vi "Main.vi"(7 "Panel":refnum<class "Panel.lvclass">, 11 "Module Admin":refnum<class "Delacor_lib_QMH_Module Admin.lvclass">) -> ()   [LabVIEW 2025, in "Chart.lvlib"]
doc: "This template is based from the Queued Message Handler design pattern and the Queued Message Handler Project Template that ships with LabVIEW 2014.\n\nThe main difference is that the Queue is private to this module and communication between modules is done via Broadcast and Request events.\n\nRequest events are wrapped via public API methods and are handled in the Event handler loop in this VI.\nAny module can register for Broadcast events sent by this module.\n\nThe Event Handling Loop generates messages based on user interface actions.\n\nThe Message Handling Loop processes messages generated by the Event Handling Loop, or by other messages. The messages are string values, so new messages can be added easily to the Message Cases case structure in the Message Handling Loop. Each message cluster can also provide an optional value for Message Data, which is a variant that can be converted to whatever message-specific data is required.\n_____\nBased on Delacor QMH Project Template 3.1.0.34.\n\n<b>Note:</b> This VI was modified by the <b>Validate DQMH Module</b> tool to call the Release Message Queue VI in the top-level Error case.\n\n<b>Note:</b> This VI was modified by the <b>Validate DQMH Module</b> tool to add a call to the Error Reported VI at the end of the 'Exit' MHL frame.\n\n<b>Note:</b> This VI was modified by the <b>Validate DQMH Module</b> tool to wrap the FP.Open method in the module close code with a Conditional Disable Structure so it does not execute when the Main VI is running as a built EXE."
uses:
  Chart.lvlib
  <vilib>/Delacor/Delacor QMH/Libraries/Module Admin_class/Delacor_lib_QMH_Module Admin.lvclass
  <vilib>/MGI/Panel Manager/Panel/Panel/Panel.lvclass
  <vilib>/Utility/miscctls.llb/LVPointTypeDef.ctl
  Module Data--cluster.ctl
  Initialise Chart Buffer Argument--cluster.ctl
  Update Chart Buffer Data Argument--cluster.ctl
  Update Chart Display Argument--cluster.ctl
  Set Chart Plot Labels Argument--cluster.ctl
  <vilib>/Delacor/Delacor QMH/Libraries/Module Admin_class/Delacor_lib_QMH_Module Admin.lvclass/Delacor_lib_QMH_Module Admin.ctl
  <vilib>/Delacor/Delacor QMH/Libraries/Message Queue_class/Delacor_lib_QMH_Message Queue.lvclass/Delacor_lib_QMH_Message Queue.ctl
  Stop Argument--cluster.ctl
  <vilib>/Delacor/Delacor QMH/Libraries/Message Queue_class/Delacor_lib_QMH_Enqueue Message (Single).vi
  <vilib>/Delacor/Delacor QMH/Libraries/Module Admin_class/Delacor_lib_QMH_Get External Launch.vi
  <vilib>/Utility/error.llb/Error Cluster From Error Code.vi
  <vilib>/ErrorRing/Error Ring.xnode
  <vilib>/Delacor/Delacor QMH/Libraries/Message Queue_class/Delacor_lib_QMH_Message Queue.lvclass
  <vilib>/MGI/Panel Manager/Panel/Panel Helper/Panel Helper.lvclass
panel:
  out "Waveform Graph":cluster{dbl, dbl, "Chart Data":dbl[][]}(graph)
  in  "Radio Buttons":enum32{"1 min", "10 min", "1 hr", "10 hr"}(radio)
  in  "Simulate MHL Error":bool
  in  "Simulate EHL Error":bool
  out "error out":errorcluster
  out "Status":string
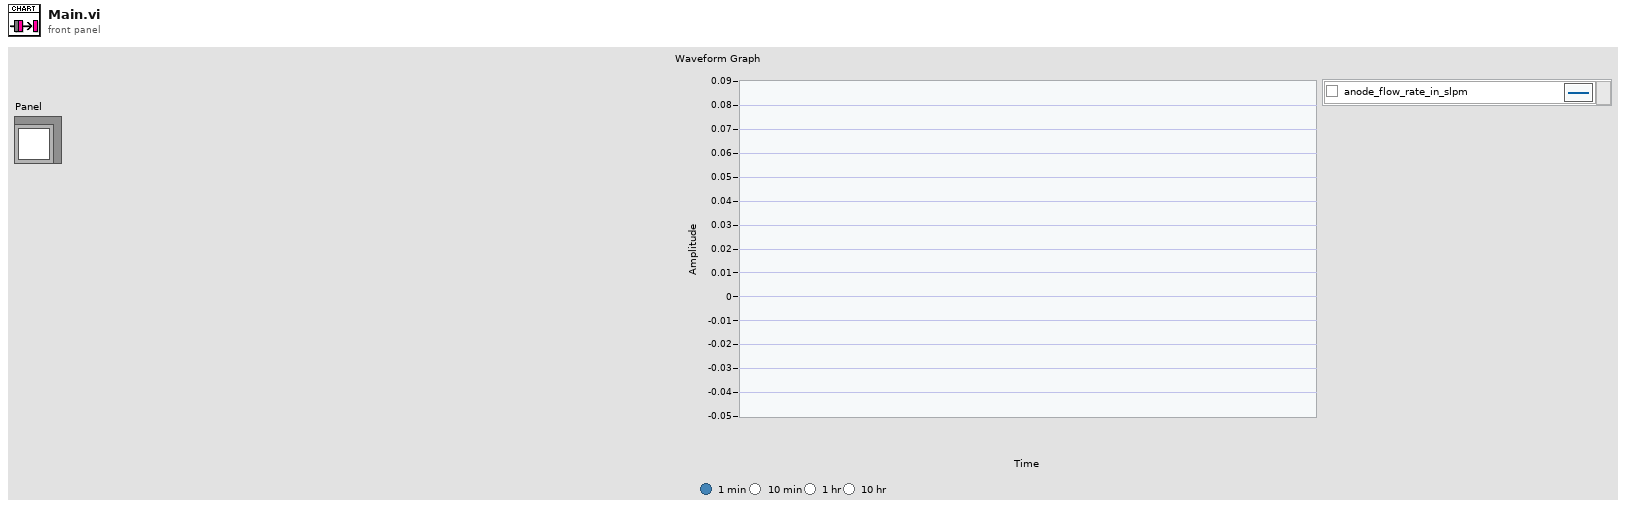
[diagram p1: front panel]
types:
  T1 = typedef "LVPointTypeDef.ctl" = cluster{"Horizontal":i16, "Vertical":i16}
  T2 = typedef "Chart.lvlib/Request Events--cluster.ctl" = cluster{"Stop Module":refnum<user-event>, "Show Panel":refnum<user-event>, "Hide Panel":refnum<user-event>, "Get Module Execution Status":refnum<user-event>, "Show Diagram":refnum<user-event>, "Change Panel":refnum<user-event>, "Initialise Chart Buffer":refnum<user-event>, "Update Chart Buffer Data":refnum<user-event>, "Update Chart Display":refnum<user-event>, "Set Chart Plot Labels":refnum<user-event>}
  T3 = typedef "Panel.lvlib/Panel Helper.lvclass/Panel Events.ctl" = cluster{"My Panel":refnum<user-event>, "Top Level Initialized":refnum<user-event>}
  T4 = typedef "Chart.lvlib/Module Data--cluster.ctl" = cluster{"Status":string, "Chart Index":i32, "Chart Data Array":dbl[][], "Frequency":dbl}
  T5 = typedef "Chart.lvlib/Stop Argument--cluster.ctl" = cluster{"Origin":string, "Exit via Stop Module Req?":bool, "Wait for Module to stop?":bool}
  T6 = typedef "Chart.lvlib/Initialise Chart Buffer Argument--cluster.ctl" = cluster{"No. of Channels":u32, "Frequency":dbl}
  T7 = typedef "Chart.lvlib/Update Chart Buffer Data Argument--cluster.ctl" = cluster{"Chart Data":dbl[]}
  T8 = typedef "Chart.lvlib/Update Chart Display Argument--cluster.ctl" = cluster{"Boolean":bool}
  T9 = typedef "Chart.lvlib/Set Chart Plot Labels Argument--cluster.ctl" = cluster{"Labels":string[]}
  T10 = enum32{"invalid lock state", "Not Locked", "Locked (No Password)", "Password-protected"}
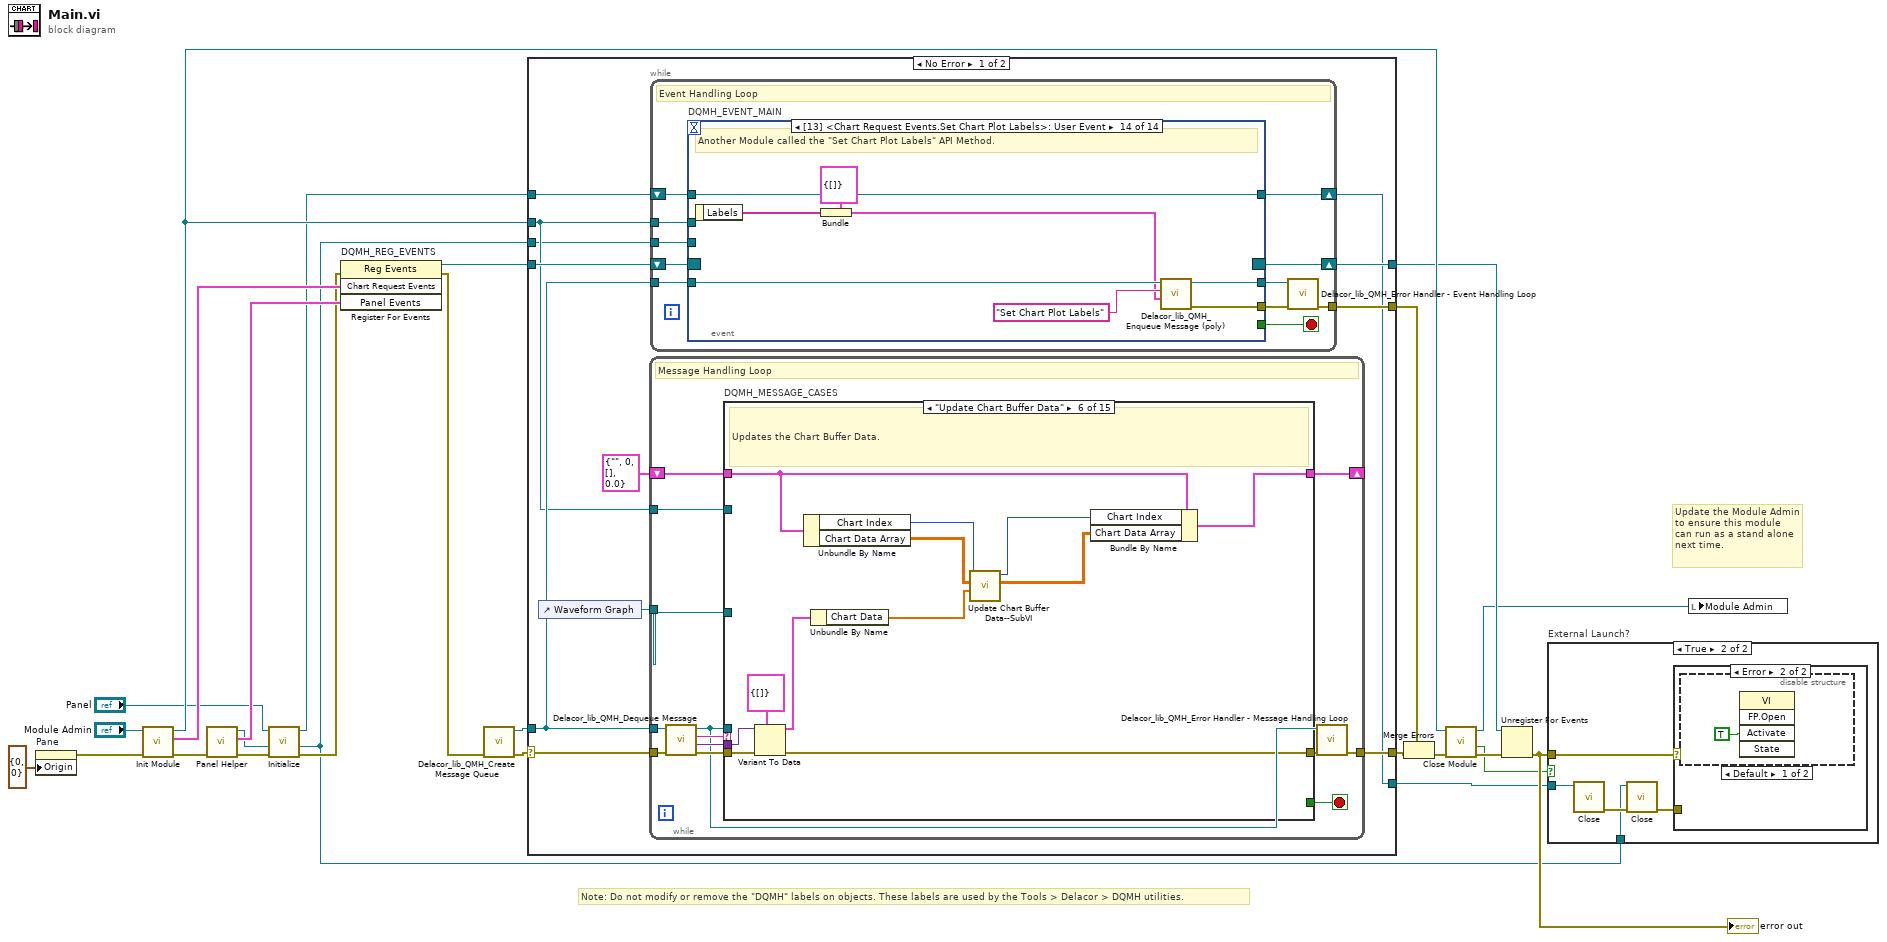
[diagram p0: block diagram]
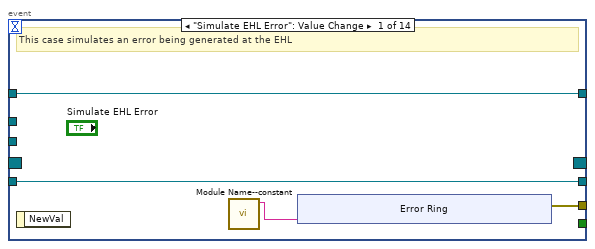
[diagram p5: hidden frame]
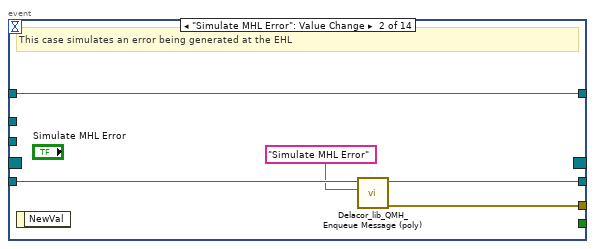
[diagram p6: hidden frame]
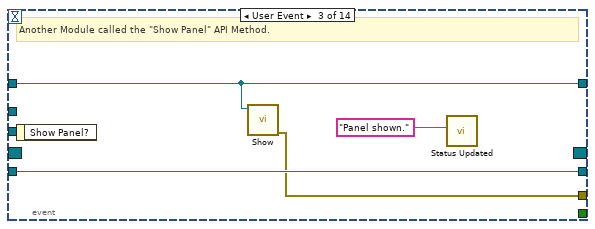
[diagram p7: hidden frame]
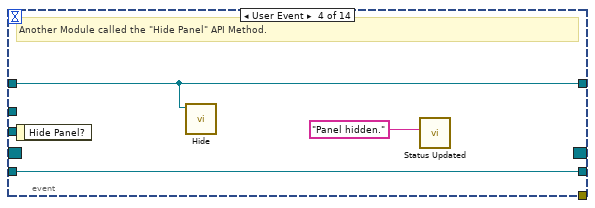
[diagram p8: hidden frame]
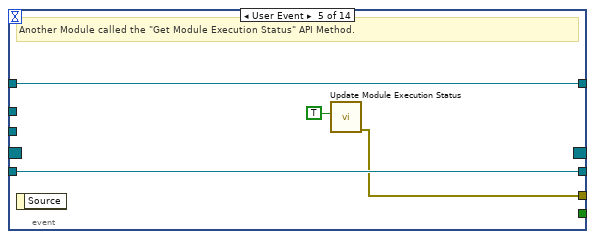
[diagram p9: hidden frame]
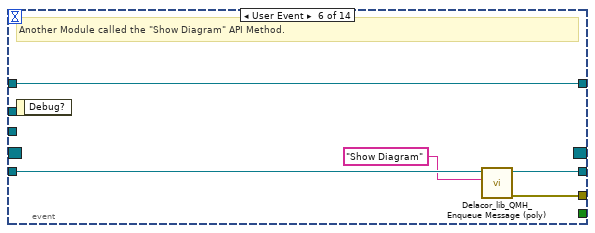
[diagram p10: hidden frame]
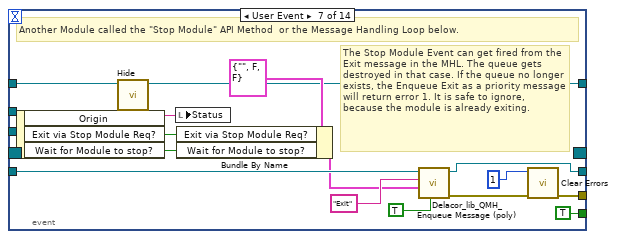
[diagram p11: hidden frame]
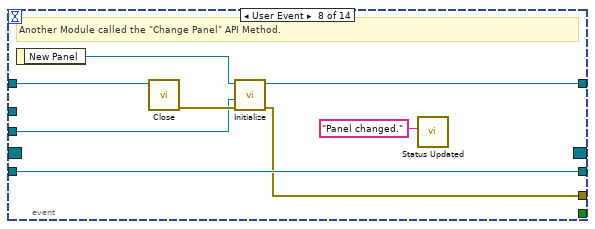
[diagram p12: hidden frame]
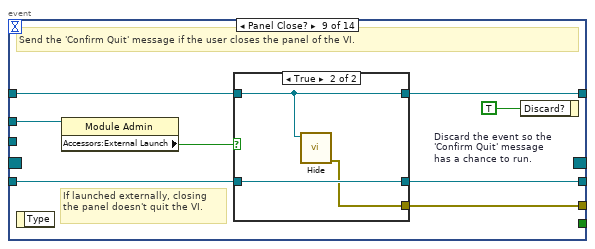
[diagram p13: hidden frame]
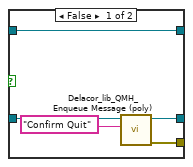
[diagram p14: hidden frame]
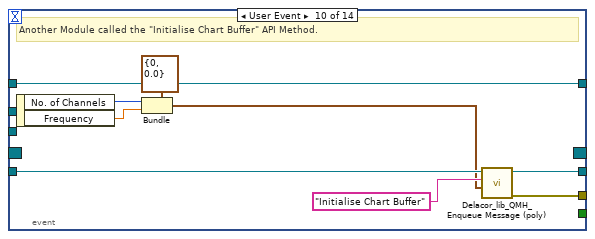
[diagram p15: hidden frame]
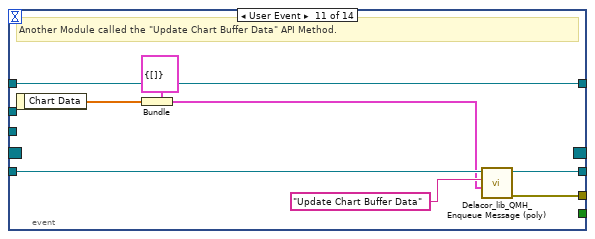
[diagram p16: hidden frame]
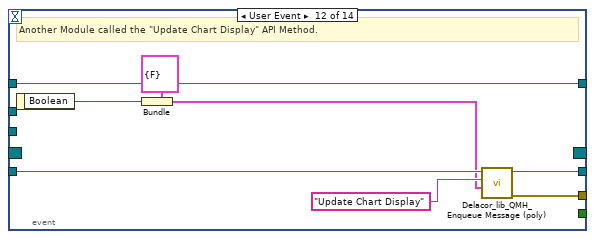
[diagram p17: hidden frame]
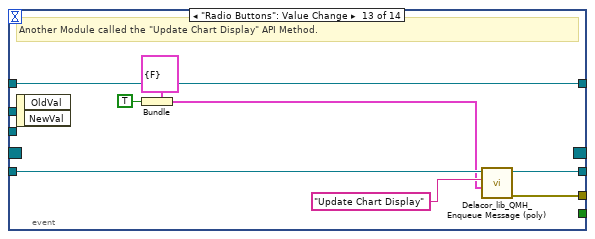
[diagram p18: hidden frame]
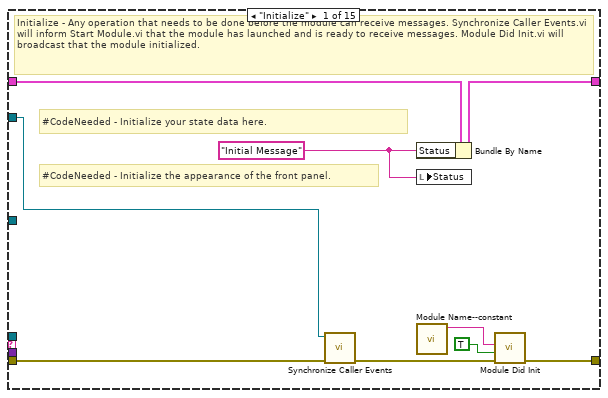
[diagram p19: hidden frame]
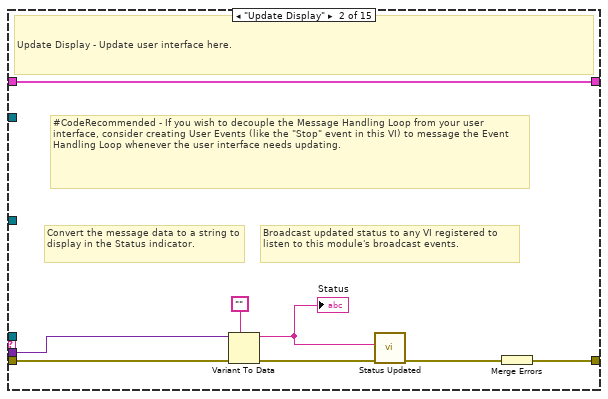
[diagram p20: hidden frame]
diagram:
  # "Note: Do not modify or remove the \"DQMH\" labels on objects. These labels are used by the Tools > Delacor > DQMH utilities."
  # "Update the Module Admin to ensure this module can run as a stand alone next time."
  n1 = property on="Pane" class="Pane"("Origin"=T1 {"Horizontal"=0, "Vertical"=0}) -> (error out=w1:errorcluster)  [unwired: 2 in, 1 out]
  n2 = call "Init Module.vi"("error in (no error)"=w1, "Singleton Module Admin in"="Module Admin") -> ("error out"=w11:errorcluster, "Chart Request Events"=w22:T2, "Singleton Module Admin out"=w26:refnum<class "Delacor_lib_QMH_Module Admin.lvclass">)  [unwired: 7 in]
  n3 = call <vilib>:"Panel Helper.vi"("Error In"=w11) -> ("Error Out"=w8:errorcluster, "Panel Events"=w10:T3, "Panel Helper out"=w7:refnum<class "Panel Helper.lvclass">)  [unwired: 8 in]
  n4 = call <vilib>:"Initialize.vi"("error in (no error)"=w8, "My Helper in"=w7, "Panel In"="Panel") -> ("error out"=w5:errorcluster, "My Helper out"=w4:refnum<class "Panel Helper.lvclass">, "Panel Out"=w3:refnum<class "Panel.lvclass">)  [unwired: 6 in]
  n5 = register-events "DQMH_REG_EVENTS"(error in=w5, w22, w10) -> (reference out=w23:refnum<event-registration>, error out=w9:errorcluster)  [unwired: 1 in]
  n6 = call <vilib>:"Delacor_lib_QMH_Create Message Queue.vi"("error in"=w9) -> ("error out"=w13:errorcluster, "Message Queue"=w21:refnum<class "Delacor_lib_QMH_Message Queue.lvclass">)  [unwired: 9 in]
  n7 = case shown="No Error" w13 {
    selector: w13 -> [w32 w363]
    tunnel: [w38 w363] -> w25
    tunnel: [w37 w368] -> w24
    tunnel: w23 -> [w35 w368]
    tunnel: w21 -> [w34 w359]
    tunnel: [w33 _] -> w17
    tunnel: w26 -> [w31 w364]
    tunnel: w3 -> [w29 w360]
    tunnel: w4 -> [w30 _]
    tunnel: [w28 w360] -> w12
    frame No Error {
      n8 = control-ref of="Waveform Graph"() -> (w27:refnum<vi>)
      n9 = while {
        tunnel: w34 -> [w165]
        shift-right: [w171] -> _
        shift-left: T4 {"Status"="", "Chart Index"=0, "Chart Data Array"=[], "Frequency"=0.0} ("Data Cluster") -> [w172]
        tunnel: w32 -> [w169]
        tunnel: [w163] -> w38
        tunnel: w31 -> [w162]
        tunnel: w27 -> [w161]
        stop <- w170 stop-if-true
        # "Message Handling Loop"
        n10 = call-dynamic "Delacor_lib_QMH_Dequeue Message.vi"("error in"=w169, "Message Queue in"=w165) -> ("error out"=w168:errorcluster, "Message Data"=w166:variant, "Message"=w167:string, "Message Queue out"=w164:refnum<class "Delacor_lib_QMH_Message Queue.lvclass">)  [unwired: 6 in]
        n11 = case "DQMH_MESSAGE_CASES" shown="\"Update Chart Buffer Data\"" w167 {
          selector: w167 -> [_ _ _ _ _ _ _ _ _ _ _ _ _ _ w348]
          tunnel: w164 -> [_ _ _ _ _ _ _ _ _ _ _ w313 w328 w344 _]
          tunnel: w168 -> [w174 w188 w192 w210 w224 w236 w256 w283 w294 w297 w302 w319 w332 w346 _]
          tunnel: [w177 w189 w191 w208 w223 w235 w255 w272 w292 w295 w300 w310 w330 w340 w349] -> w173
          tunnel: w172 -> [w182 w190 w193 w209 w212 w229 w242 w282 w293 w296 w301 w318 w331 w343 w350]
          tunnel: [w181 w190 w193 w209 w211 w228 w242 w282 w293 w296 w301 w318 w331 w343 w350] -> w171
          tunnel: [_ _ _ _ _ _ _ _ _ _ _ _ _ w342 _] -> w170
          tunnel: w166 -> [_ w187 _ _ w222 w234 w254 w281 _ _ _ w317 _ w339 _]
          tunnel: w162 -> [w175 _ _ _ _ _ _ _ _ _ _ w312 _ w333 _]
          tunnel: w161 -> [_ _ _ _ _ _ w237 w269 _ _ _ _ _ _ _]
          frame "Initialize" {
            w180 = "Initial Message" ("Initial Message")
            # "#CodeNeeded - Initialize the appearance of the front panel."
            # "#CodeNeeded - Initialize your state data here."
            # "Initialize - Any operation that needs to be done before the module can receive messages. Synchronize Caller Events.vi will inform Start Module.vi that the module has launched and is ready to receive messages. Module Did Init.vi will broadcast that the module initialized."
            n12 = call "Synchronize Caller Events.vi"("error in (no error)"=w174, "Singleton Module Admin in"=w175) -> ("error out"=w176:errorcluster)  [unwired: 8 in, 1 out]
            n13 = Bundle By Name(cluster=w182, "Status"=w180) -> (w181:T4)
            n14 = local write "Status"(w180) -> ()
            n15 = call "Module Name--constant.vi"() -> ("Module Name"=w178:string)  [unwired: 11 in]
            n16 = call "Module Did Init.vi"("error in (no error)"=w176, "Initialized?"=TRUE, "Origin"=w178) -> ("error out"=w177:errorcluster)  [unwired: 8 in]
          }
          frame "Update Display" {
            # "Broadcast updated status to any VI registered to listen to this module's broadcast events."
            # "Convert the message data to a string to display in the Status indicator."
            # "#CodeRecommended - If you wish to decouple the Message Handling Loop from your user interface, consider creating User Events (like the \"Stop\" event in this VI) to message the Event Handling Loop whenever the user interface needs updating."
            # "Update Display - Update user interface here."
            n17 = Variant To Data(error in=w188, type="" ("Empty String Constant"), Variant=w187) -> (data=w185:string, error out=w184:errorcluster)
            "Status" <- w185
            n18 = call "Status Updated.vi"("error in (no error)"=w184, "Status"=w185) -> ("error out"=w183:errorcluster)  [unwired: 9 in]
            n19 = Merge Errors(w183) -> (w189:errorcluster)
          }
          frame "Show Diagram" {
            # "Show Diagram - Show the block diagram of this VI. Used as a debugging tool. There is a button in the module tester that fires the Show Diagram request, which runs this message. Note that the diagram will not be displayed if it is password-protected and the password is not in the cache."
            n20 = disable-structure shown="RUN_TIME_ENGINE==False" {
              disable-tunnel: [w201 w207] -> w191
              disable-tunnel: w192 -> [w200 w207]
              frame condition #0 (active) {
                # "functionality not available in exe"
                n21 = invoke on="Invoke Node" class="VI" method="Lock State.Get"(error in=w200) -> (error out=w199:errorcluster, "Get Lock State"=w198:T10, "pwd in cache"=w195:bool)  [unwired: 3 in, 1 out]
                n22 = Equal?(x=T10."Password-protected", y=w198) -> (x = y?=w196:bool)
                n23 = Compound Arithmetic op=AND(w196, invert w195) -> (w194:bool)
                n24 = case shown="False" w194 {
                  tunnel: [w204 w206] -> w201
                  tunnel: w199 -> [w202 w206]
                  frame False {
                    n25 = property on="Property Node" class="VI"(error in=w202, "BDWin.Open"=TRUE ("Block Diagram Window:Open")) -> (error out=w204:errorcluster)  [unwired: 1 in, 1 out]
                    n26 = call "Status Updated.vi"("Status"="Block Diagram shown." ("format string")) -> ()  [unwired: 10 in, 1 out]
                  }
                  frame True {
                    # "Password-protected VI, and the password is not in the cache. Do not show the diagram."
                  }
                }
              }
              frame condition #1 {
              }
            }
          }
          frame "--- Module Specific ---" {
            # "Separator -- The following cases handle messages specific to this Module."
            n27 = Merge Errors(w210) -> (w208:errorcluster)
          }
          frame "Initialise Chart Buffer" {
            # "Initialises the chart buffer."
            n28 = Variant To Data(error in=w224, type=T6 {"No. of Channels"=0, "Frequency"=0.0} ("Initialise Chart Buffer Argument"), Variant=w222) -> (data=w213:T6, error out=w223:errorcluster)
            n29 = Unbundle By Name(w213) -> ("No. of Channels"=w215:u32, "Frequency"=w216:dbl)
            n30 = Multiply(x=w216, y=36000.0) -> (x*y=w214:dbl)
            n31 = Initialize Array(nan ("element"), w215, w214) -> (w217:dbl[][])
            n32 = Bundle By Name(cluster=w212, "Chart Index"=0, "Chart Data Array"=w217, "Frequency"=w216) -> (w211:T4)
          }
          frame "Update Chart Buffer Data" {
            # "Updates the Chart Buffer Data."
            n33 = Variant To Data(error in=w236, type=T7 {"Chart Data"=[]} ("Update Chart Buffer Data Argument"), Variant=w234) -> (data=w232:T7, error out=w235:errorcluster)
            n34 = Unbundle By Name(w229) -> ("Chart Index"=w226:i32, "Chart Data Array"=w231:dbl[][])
            n35 = Unbundle By Name(w232) -> ("Chart Data"=w230:dbl[])
            n36 = call "Update Chart Buffer Data--SubVI.vi"("Chart Data"=w230, "Chart Buffer In"=w231, "Chart Index In"=w226) -> ("Chart Buffer Out"=w227:dbl[][], "Chart Index Out"=w225:i32)  [unwired: 7 in]
            n37 = Bundle By Name(cluster=w229, "Chart Index"=w225, "Chart Data Array"=w227) -> (w228:T4)
          }
          frame "Update Chart Display" {
            # "Updates the Chart Display."
            n38 = Unbundle By Name(w242) -> ("Chart Data Array"=w246:dbl[][], "Chart Index"=w252:i32, "Frequency"=w250:dbl)
            n39 = Variant To Data(error in=w256, type=T8 {"Boolean"=FALSE} ("Update Chart Display Argument"), Variant=w254) -> (error out=w255:errorcluster)  [unwired: 1 out]
            n40 = Get Date/Time In Seconds() -> (seconds since 1Jan1904=w251:timestamp)
            n41 = case shown="\"10 hr\"" "Radio Buttons" {
              tunnel: w250 -> [w259 w262 w265 w268]
              tunnel: [w258 w261 w264 w267] -> w245
              tunnel: [w257 w260 w263 w266] -> w247
              frame "1 min", Default {
                w257 = 60.0 ("y")
                n42 = Multiply(x=w259, y=w257) -> (x*y=w258:dbl)
              }
              frame "10 min" {
                w260 = 600.0 ("y")
                n43 = Multiply(x=w262, y=w260) -> (x*y=w261:dbl)
              }
              frame "1 hr" {
                w263 = 3600.0 ("y")
                n44 = Multiply(x=w265, y=w263) -> (x*y=w264:dbl)
              }
              frame "10 hr" {
                w266 = 36000.0 ("y")
                n45 = Multiply(x=w268, y=w266) -> (x*y=w267:dbl)
              }
            }
            n46 = To Double Precision Float(number=w251) -> (double precision float=w249:dbl)
            n47 = Subtract(x=w249, y=w247) -> (x-y=w248:dbl)
            n48 = Subtract(x=w252, y=w245) -> (x-y=w243:dbl)
            n49 = property on="Property Node" class="WFGraph (strict)"(reference=w237, "XScale.Offset"=w248) -> ()  [unwired: 1 in, 2 out]
            n50 = call "Update Chart Display--SubVI.vi"("Length"=w245, "Start Index"=w243, "Chart Data Array"=w246) -> ("Chart Data"=w244:dbl[][])  [unwired: 8 in]
            n51 = Bundle(0.0, 1.0, "Chart Data"=w244) -> (→"Waveform Graph":cluster{dbl, dbl, "Chart Data":dbl[][]})  [unwired: 1 in]
          }
          frame "Set Chart Plot Labels" {
            # "Set Chart Plot Labels."
            n52 = Variant To Data(error in=w283, type=T9 {"Labels"=[]} ("Set Chart Plot Labels Argument"), Variant=w281) -> (data=w279:T9, error out=w273:errorcluster)
            n53 = Unbundle By Name(w279) -> ("Labels"=w270:string[])
            n54 = for {
              tunnel: w270 -> [w291] mode=indexing
              tunnel: [w285] -> w274
              tunnel: errorcluster {"status"=FALSE, "code"=0, "source"=""} ("error out") -> [w288]
              tunnel: [w289] -> w276
              shift-right: [w290] -> w278
              shift-left: w269 -> [w284]
              i -> [w285]
              # "Only show 1st 3 plots"
              n55 = Less?(x=w285, y=3) -> (x < y?=w286:bool)
              n56 = property on="Property Node" class="WFGraph (strict)"(reference=w284, error in=w288, "Active Plot"=w285, "Plot.Plot Name"=w291, "Plot.Visible?"=w286) -> (reference out=w290:refnum<vi>, error out=w289:errorcluster)
            }
            n57 = property on="Property Node" class="WFGraph (strict)"(reference=w278, error in=w276, "LegAutosize"=FALSE ("Legend:Autosize"), "LegNumRows"=w274) -> (error out=w275:errorcluster)  [unwired: 1 out]
            n58 = Merge Errors(w275, w273) -> (w272:errorcluster)
          }
          frame "---Copy This Frame---" {
            # "Duplicate this frame when creating new messages.  Change this comment in the duplicated frame to describe this message."
            n59 = Merge Errors(w294) -> (w292:errorcluster)
          }
          frame "--- Exit and Error Handling---" {
            # "Separator - The following cases handle errors and exit messages."
            n60 = Merge Errors(w297) -> (w295:errorcluster)
          }
          frame "Simulate MHL Error" {
            # "Simulate an error occurring at the MHL"
            n61 = call "Module Name--constant.vi"() -> ("Module Name"=w299:string)  [unwired: 11 in]
            n62 = xnode "Error Ring"("parameter 0"=w299) -> ("error out"=w298:errorcluster)
            n63 = Merge Errors(w302, w298) -> (w300:errorcluster)
          }
          frame "Error" {
            # "#CodeRecommended - If you ever change the name of this \"Error\" message, you'll need to update the name in the Check Loop Error.vi as well."
            # "#CodeRecommended - If the module is running in standalone mode (External Launch = FALSE), this code will pop up an error dialog and call the 'Exit' message if an error occurs. Add more fine-grained error handling here."
            # "Error - Check the error message data and respond accordingly. This message is sent by the \"Error Handler\" VIs at the end of each loop in this application."
            n64 = property on="Property Node" class="Module Admin"(reference=w312) -> ("Accessors:External Launch"=w311:bool)  [unwired: 1 in, 2 out]
            n65 = Variant To Data(error in=w319, type=errorcluster {"status"=FALSE, "code"=0, "source"=""} ("error constant"), Variant=w317) -> (data=w320:errorcluster, error out=w315:errorcluster)
            n66 = call "Error Reported.vi"("Error"=w320) -> ()  [unwired: 10 in, 1 out]
            n67 = case shown="False" w311 {
              tunnel: [w325 _] -> w314
              tunnel: w313 -> [w324 _]
              tunnel: w320 -> [w321 _]
              frame False {
                # "If the module is running standalone, then pop up an error dialog and call the \"Exit\" message."
                n68 = call <vilib>:"Simple Error Handler.vi"("error in (no error)"=w321) -> ()  [unwired: 4 in, 5 out]
                n69 = call-poly <vilib>:"Delacor_lib_QMH_Enqueue Message (poly).vi"("Priority Message? (F)"=TRUE, "Message"="Exit", "Message Queue in"=w324) -> ("error out"=w325:errorcluster)  [unwired: 7 in, 1 out]
              }
              frame True {
                # "If the module was launched externally, calling the Error Reported broadcast VI is the only action performed by the \"Error\" message. The module's caller can then process the error appropriately."
              }
            }
            n70 = Merge Errors(w315, w314) -> (w310:errorcluster)
            n71 = local write "error out"(w310) -> ()
          }
          frame "Confirm Quit" {
            # "#CodeNeeded - If you want to provide an \"Are you sure\" dialog (or some other notification) before the application exits, place that code here. This message is typically sent from a Panel Close? event."
            # "Confirm Quit - Message that can confirm whether or not the user wants to exit the application."
            n72 = call-poly <vilib>:"Delacor_lib_QMH_Enqueue Message (poly).vi"("Priority Message? (F)"=TRUE, "error in"=w332, "Message"="Exit", "Message Queue in"=w328) -> ("error out"=w329:errorcluster)  [unwired: 6 in, 1 out]
            n73 = Merge Errors(w329) -> (w330:errorcluster)
          }
          frame "Exit" {
            w337 = 91  # 91: not all Exit messages will have an argument
            w342 = TRUE  # Stop the VI
            # "Release the message queue reference"
            # "#CodeNeeded - Add any required cleanup code here"
            # "Exit - Exit the application."
            n74 = Variant To Data(error in=w346, type=T5 {"Origin"="", "Exit via Stop Module Req?"=FALSE, "Wait for Module to stop?"=FALSE} ("Stop Argument"), Variant=w339) -> (data=w335:T5, error out=w338:errorcluster)
            n75 = call <vilib>:"Clear Errors.vi"("error in (no error)"=w338, "specific error code to clear (0: all)"=w337) -> ("error out"=w345:errorcluster)  [unwired: 4 in, 1 out]
            n76 = call-dynamic "Delacor_lib_QMH_Release Message Queue.vi"("error in"=w345, "Message Queue"=w344) -> ("error out"=w341:errorcluster)  [unwired: 9 in]
            n77 = call "Handle Exit.vi"("Stop Argument"=w335, "Admin in"=w333) -> ("error out"=w334:errorcluster)  [unwired: 8 in, 1 out]
            n78 = Merge Errors(w334, w341) -> (w340:errorcluster)
            n79 = call "Error Reported.vi"("Error"=w340) -> ()  [unwired: 10 in, 1 out]
          }
          frame Default {
            # "'Default' case only runs if there is a message that isn't defined in any of the other cases.  Output a programming error."
            n80 = call "Module Name--constant.vi"() -> ("Module Name"=w347:string)  [unwired: 11 in]
            n81 = xnode "Error Ring"("parameter 0"=w348, "parameter 1"=w347) -> ("error out"=w349:errorcluster)
          }
        }
        n82 = call-dynamic "Delacor_lib_QMH_Error Handler - Message Handling Loop.vi"("error in"=w173, "Message Queue in"=w164) -> ("dup error in"=w163:errorcluster)  [unwired: 8 in, 1 out]
      }
      n83 = while {
        tunnel: w34 -> [w49]
        shift-right: [w47] -> w37
        shift-left: w35 -> [w48]
        tunnel: [w43] -> w33
        tunnel: w31 -> [w42]
        tunnel: w30 -> [w41]
        shift-right: [w39] -> w28
        shift-left: w29 -> [w40]
        stop <- w45 stop-if-true
        # "Event Handling Loop"
        n84 = event "DQMH_EVENT_MAIN" shown="[13] <Chart Request Events.Set Chart Plot Labels>: User Event" {
          selector: w48 -> [_ _ _ _ _ _ _ _ _ _ _ _ _ _]
          dyn-events: [_ _ _ _ _ _ _ _ _ _ _ _ _ _] -> w47
          timeout: _ -> [_ _ _ _ _ _ _ _ _ _ _ _ _ _]
          tunnel: [_ _ _ _ _ _ TRUE ("Discard?") _ _ _ _ _ _ _] -> w45
          tunnel: w49 -> [w53 w65 w69 w72 w76 w81 w93 w103 w110 w128 w136 w144 w152 w160]
          tunnel: [w52 w62 w67 _ w75 w78 w87 w99 w109 w120 w129 w137 w146 w153] -> w46
          tunnel: [w53 w64 w69 w72 w76 w80 w92 w103 w108 w126 w134 w142 w150 w158] -> w44
          tunnel: w42 -> [_ _ _ _ _ _ _ _ w107 _ _ _ _ _]
          tunnel: w41 -> [_ _ _ _ _ _ _ w98 _ _ _ _ _ _]
          tunnel: w40 -> [w50 w61 w68 w71 w73 w77 w82 w102 w105 w127 w135 w143 w151 w159]
          tunnel: [w50 w61 w68 w71 w73 w77 w82 w97 w104 w127 w135 w143 w151 w159] -> w39
          event "Simulate EHL Error": Value Change {
            # "This case simulates an error being generated at the EHL"
            n85 = event-data() -> ()  [unwired: 1 in, 1 out]
            n86 = call "Module Name--constant.vi"() -> ("Module Name"=w51:string)  [unwired: 11 in]
            n87 = xnode "Error Ring"("parameter 0"=w51) -> ("error out"=w52:errorcluster)
          }
          event "Simulate MHL Error": Value Change {
            # "This case simulates an error being generated at the EHL"
            n88 = event-data() -> ()  [unwired: 1 in, 1 out]
            n89 = call-poly <vilib>:"Delacor_lib_QMH_Enqueue Message (poly).vi"("Message"="Simulate MHL Error", "Message Queue in"=w65) -> ("error out"=w62:errorcluster, "Message Queue out"=w64:refnum<class "Delacor_lib_QMH_Message Queue.lvclass">)  [unwired: 8 in]
          }
          event User Event {
            # "Another Module called the \"Show Panel\" API Method."
            n90 = event-data() -> ()  [unwired: 1 in, 1 out]
            n91 = call <vilib>:"Show.vi"("Panel in"=w68) -> ("Error Out"=w67:errorcluster)  [unwired: 10 in]
            n92 = call "Status Updated.vi"("Status"="Panel shown." ("format string")) -> ()  [unwired: 10 in, 1 out]
          }
          event User Event {
            # "Another Module called the \"Hide Panel\" API Method."
            n93 = event-data() -> ()  [unwired: 1 in, 1 out]
            n94 = call <vilib>:"Hide.vi"("Panel In"=w71) -> ()  [unwired: 10 in, 1 out]
            n95 = call "Status Updated.vi"("Status"="Panel hidden." ("format string")) -> ()  [unwired: 10 in, 1 out]
          }
          event User Event {
            # "Another Module called the \"Get Module Execution Status\" API Method."
            n96 = event-data() -> ()  [unwired: 1 in, 1 out]
            n97 = call "Update Module Execution Status.vi"("Running?"=TRUE) -> ("error out"=w75:errorcluster)  [unwired: 10 in]
          }
          event User Event {
            # "Another Module called the \"Show Diagram\" API Method."
            n98 = event-data() -> ()  [unwired: 1 in, 1 out]
            n99 = call-poly <vilib>:"Delacor_lib_QMH_Enqueue Message (poly).vi"("Message"="Show Diagram", "Message Queue in"=w81) -> ("error out"=w78:errorcluster, "Message Queue out"=w80:refnum<class "Delacor_lib_QMH_Message Queue.lvclass">)  [unwired: 8 in]
          }
          event User Event {
            # "The Stop Module Event can get fired from the Exit message in the MHL. The queue gets destroyed in that case. If the queue no longer exists, the Enqueue Exit as a priority message will return error 1. It is safe to ignore, because the module is already exiting."
            # "Another Module called the \"Stop Module\" API Method  or the Message Handling Loop below."
            n100 = event-data() -> ("Origin"=w91:string, "Exit via Stop Module Req?"=w85:bool, "Wait for Module to stop?"=w84:bool)  [unwired: 1 in]
            n101 = call <vilib>:"Hide.vi"("Panel In"=w82) -> ()  [unwired: 10 in, 1 out]
            n102 = local write "Status"(w91) -> ()
            n103 = Bundle By Name(cluster=T5 {"Origin"="", "Exit via Stop Module Req?"=FALSE, "Wait for Module to stop?"=FALSE} ("Stop Argument"), "Exit via Stop Module Req?"=w85, "Wait for Module to stop?"=w84) -> (w83:T5)
            n104 = call-poly <vilib>:"Delacor_lib_QMH_Enqueue Message (poly).vi"("Priority Message? (F)"=TRUE, "Message Data"=w83, "Message"="Exit", "Message Queue in"=w93) -> ("error out"=w88:errorcluster, "Message Queue out"=w92:refnum<class "Delacor_lib_QMH_Message Queue.lvclass">)  [unwired: 6 in]
            n105 = call <vilib>:"Clear Errors.vi"("error in (no error)"=w88, "specific error code to clear (0: all)"=1) -> ("error out"=w87:errorcluster)  [unwired: 4 in, 1 out]
          }
          event User Event {
            # "Another Module called the \"Change Panel\" API Method."
            n106 = event-data() -> ("New Panel"=w101:refnum<class "Panel.lvclass">)  [unwired: 1 in]
            n107 = call-dynamic <vilib>:"Close.vi"("Panel In"=w102) -> ("Error Out"=w100:errorcluster)  [unwired: 10 in]
            n108 = call <vilib>:"Initialize.vi"("error in (no error)"=w100, "My Helper in"=w98, "Panel In"=w101) -> ("error out"=w99:errorcluster, "Panel Out"=w97:refnum<class "Panel.lvclass">)  [unwired: 6 in, 1 out]
            n109 = call "Status Updated.vi"("Status"="Panel changed.") -> ()  [unwired: 10 in, 1 out]
          }
          event Panel Close? {
            w111 = TRUE  # Discard the event so the 'Confirm Quit' message has a chance to run.
            # "If launched externally, closing the panel doesn't quit the VI."
            # "Send the 'Confirm Quit' message if the user closes the panel of the VI."
            n110 = event-data() -> ()  [unwired: 1 in, 1 out]
            n111 = property on="Property Node" class="Module Admin"(reference=w107) -> ("Accessors:External Launch"=w106:bool)  [unwired: 1 in, 2 out]
            n112 = case shown="True" w106 {
              tunnel: w110 -> [w116 w119]
              tunnel: [w115 w117] -> w109
              tunnel: [w114 w119] -> w108
              tunnel: w105 -> [w112 w118]
              tunnel: [w112 w118] -> w104
              frame False {
                n113 = call-poly <vilib>:"Delacor_lib_QMH_Enqueue Message (poly).vi"("Message"="Confirm Quit", "Message Queue in"=w116) -> ("error out"=w115:errorcluster, "Message Queue out"=w114:refnum<class "Delacor_lib_QMH_Message Queue.lvclass">)  [unwired: 8 in]
              }
              frame True {
                n114 = call <vilib>:"Hide.vi"("Panel In"=w118) -> ("Error Out"=w117:errorcluster)  [unwired: 10 in]
              }
            }
            n115 = event-data ("Event Filter Node")("Discard?"=w111) -> ()  [unwired: 1 in, 1 out]
          }
          event User Event {
            # "Another Module called the \"Initialise Chart Buffer\" API Method."
            n116 = event-data() -> ("No. of Channels"=w122:u32, "Frequency"=w121:dbl)  [unwired: 1 in]
            n117 = Bundle(cluster=T6 {"No. of Channels"=0, "Frequency"=0.0} ("Initialise Chart Buffer Argument"), "No. of Channels"=w122, "Frequency"=w121) -> (w123:T6)
            n118 = call-poly <vilib>:"Delacor_lib_QMH_Enqueue Message (poly).vi"("Message Data"=w123, "Message"="Initialise Chart Buffer", "Message Queue in"=w128) -> ("error out"=w120:errorcluster, "Message Queue out"=w126:refnum<class "Delacor_lib_QMH_Message Queue.lvclass">)  [unwired: 7 in]
          }
          event User Event {
            # "Another Module called the \"Update Chart Buffer Data\" API Method."
            n119 = event-data() -> ("Chart Data"=w130:dbl[])  [unwired: 1 in]
            n120 = Bundle(cluster=T7 {"Chart Data"=[]} ("Update Chart Buffer Data Argument"), "Chart Data"=w130) -> (w131:T7)
            n121 = call-poly <vilib>:"Delacor_lib_QMH_Enqueue Message (poly).vi"("Message Data"=w131, "Message"="Update Chart Buffer Data", "Message Queue in"=w136) -> ("error out"=w129:errorcluster, "Message Queue out"=w134:refnum<class "Delacor_lib_QMH_Message Queue.lvclass">)  [unwired: 7 in]
          }
          event User Event {
            # "Another Module called the \"Update Chart Display\" API Method."
            n122 = event-data() -> ("Boolean"=w138:bool)  [unwired: 1 in]
            n123 = Bundle(cluster=T8 {"Boolean"=FALSE} ("Update Chart Display Argument"), "Boolean"=w138) -> (w139:T8)
            n124 = call-poly <vilib>:"Delacor_lib_QMH_Enqueue Message (poly).vi"("Message Data"=w139, "Message"="Update Chart Display", "Message Queue in"=w144) -> ("error out"=w137:errorcluster, "Message Queue out"=w142:refnum<class "Delacor_lib_QMH_Message Queue.lvclass">)  [unwired: 7 in]
          }
          event "Radio Buttons": Value Change {
            # "Another Module called the \"Update Chart Display\" API Method."
            n125 = event-data() -> ()  [unwired: 1 in, 2 out]
            n126 = Bundle(cluster=T8 {"Boolean"=FALSE} ("Update Chart Display Argument"), "Boolean"=TRUE) -> (w147:T8)
            n127 = call-poly <vilib>:"Delacor_lib_QMH_Enqueue Message (poly).vi"("Message Data"=w147, "Message"="Update Chart Display", "Message Queue in"=w152) -> ("error out"=w146:errorcluster, "Message Queue out"=w150:refnum<class "Delacor_lib_QMH_Message Queue.lvclass">)  [unwired: 7 in]
          }
          event User Event {
            # "Another Module called the \"Set Chart Plot Labels\" API Method."
            n128 = event-data() -> ("Labels"=w154:string[])  [unwired: 1 in]
            n129 = Bundle(cluster=T9 {"Labels"=[]} ("Set Chart Plot Labels Argument"), "Labels"=w154) -> (w155:T9)
            n130 = call-poly <vilib>:"Delacor_lib_QMH_Enqueue Message (poly).vi"("Message Data"=w155, "Message"="Set Chart Plot Labels", "Message Queue in"=w160) -> ("error out"=w153:errorcluster, "Message Queue out"=w158:refnum<class "Delacor_lib_QMH_Message Queue.lvclass">)  [unwired: 7 in]
          }
        }
        n131 = call-dynamic "Delacor_lib_QMH_Error Handler - Event Handling Loop.vi"("error in"=w46, "Message Queue in"=w44) -> ("dup error in"=w43:errorcluster)  [unwired: 8 in, 1 out]
      }
    }
    frame Error {
      # "Synchronize Caller Events.vi will inform Start Module.vi that the module has launched and will let the code calling Start Module.vi register for broadcasts and would permit the caller receive the broadcast that an error occurred at launch time."
      n132 = call-dynamic "Delacor_lib_QMH_Release Message Queue.vi"("Message Queue"=w359) -> ()  [unwired: 10 in, 1 out]
      n133 = call "Synchronize Caller Events.vi"("Singleton Module Admin in"=w364) -> ("error out"=w361:errorcluster)  [unwired: 9 in, 1 out]
      n134 = call "Module Name--constant.vi"() -> ("Module Name"=w367:string)  [unwired: 11 in]
      n135 = Format Into String(format string="An error occurred during initialization. %s is no longer running.", w367) -> (resulting string=w365:string)  [unwired: 2 in, 1 out]
      n136 = Merge Errors(w363, w361) -> (w362:errorcluster)
      n137 = call "Error Reported.vi"("Additional Information"=w365, "Error"=w362) -> ()  [unwired: 9 in, 1 out]
    }
  }
  n138 = Merge Errors(w17, w25) -> (w16:errorcluster)
  n139 = call "Close Module.vi"("error in (no error)"=w16, "Module Admin in"=w26) -> ("error out"=w19:errorcluster, "External Launch"=w14:bool, "Module Admin out"=w18:refnum<class "Delacor_lib_QMH_Module Admin.lvclass">)  [unwired: 7 in]
  n140 = Unregister For Events(event registration refnum=w24, error in=w19) -> (error out=w15:errorcluster)
  "error out" <- w15
  n141 = case "External Launch?" shown="True" w14 {
    tunnel: w15 -> [_ w373]
    tunnel: w12 -> [_ w372]
    tunnel: w4 -> [_ w370]
    frame False {
    }
    frame True {
      n142 = call-dynamic <vilib>:"Close.vi"("Panel In"=w372) -> ("Error Out"=w371:errorcluster)  [unwired: 10 in]
      n143 = call <vilib>:"Close.vi"("error in (no error)"=w371, "Controller in"=w370) -> ("error out"=w369:errorcluster)  [unwired: 9 in]
      n144 = case shown="Error" w373 {
        tunnel: w369 -> [_ _]
        frame No Error {
        }
        frame Error {
          n145 = disable-structure shown="Default" {
            frame condition #0 (active) {
              n146 = invoke class="VI" method="FP.Open"("Activate"=TRUE ("Activate?")) -> ()  [unwired: 4 in, 5 out]
            }
            frame condition #1 {
              # "Don't show panel on error if running inside a built EXE."
            }
          }
        }
      }
    }
  }
  n147 = local write "Module Admin"(w18) -> ()
